vi "Interpolation.vi"(1 "Start Distance":dbl=60.0 format="%#_13g", 2 "Current Ultrasonic Distance":dbl) -> (0 "Motor Output":dbl)   [LabVIEW 2017]
panel:
  # "Interpolation\nTeam 34 Rockets"
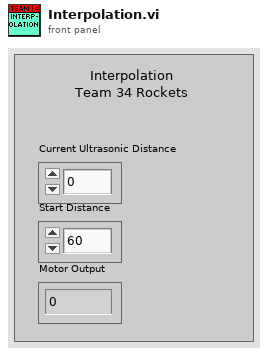
[diagram p1: front panel]
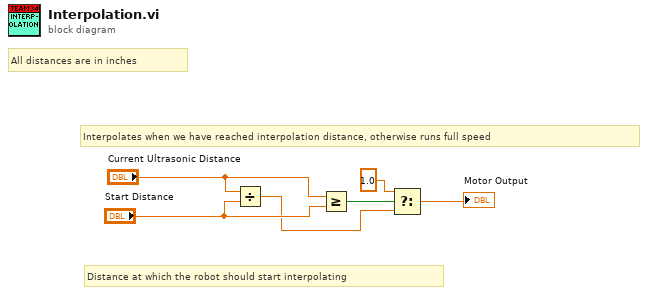
[diagram p0: block diagram]
diagram:
  # "All distances are in inches"
  # "Interpolates when we have reached interpolation distance, otherwise runs full speed"
  # "Distance at which the robot should start interpolating"
  n1 = Divide(x="Current Ultrasonic Distance", y="Start Distance") -> (x/y=w1:dbl)
  n2 = Greater Or Equal?(x="Current Ultrasonic Distance", y="Start Distance") -> (x >= y?=w4:bool)
  n3 = Select(t=1.0, s=w4, f=w1) -> (s? t:f=→"Motor Output":dbl)
